vi "methodeändern-15-07-17.vi"(2 "->Methode":T2, 3 "Namen":T3) -> (1 "Methode->":T1)   [LabVIEW 2010]
panel:
  in  "T_MainMach2":dbl[](array[numeric])
  in  "t_MainMach2":dbl[](array[numeric])
  in  "T_MainMach1":dbl[](array[numeric])
  in  "t_MainMach1":dbl[](array[numeric])
  out "Methode":string
  in  "Int.Stop2":dbl
  in  "Int.Start2":dbl
  in  "Int.Stop1":dbl
  in  "Int.Start1":dbl
  in  "ZeitpktMS-2":dbl
  in  "ZeitpktMS-1":dbl
  in  "SetpointMPV":i32[](array[numeric]) min=1 max=6 step=1
  in  "ZeitpunkteMPV":dbl[](array[numeric])
  in  "Editor verlassen":bool
  out "langsameHeizungen":string[](array[string])
  out "HorstSPMod2B":string[](array[string])
  out "HorstSPMod2A":string[](array[string])
  out "HorstSPMod1":string[](array[string])
  out "HorstSPMod0":string[](array[string])
  out "DIOsSPMod0":string[](array[string])
  out "DIOsSPMod2A":string[](array[string])
  out "DIOsSPMod2B":string[](array[string])
  out "DIOsSPMod1":string[](array[string])
  in  "Zykluslängen [s]":dbl[](array[numeric])
  in  "MS-Daten?":bool
  in  "PIDs für \"träge\" Heizungen":T4(array[cluster])
  in  "T_PreMach2":dbl[](array[numeric])
  in  "t_PreMach2":dbl[](array[numeric])
  in  "T_PreMach1":dbl[](array[numeric])
  in  "t_PreMach1":dbl[](array[numeric])
  in  "FPGAFixp":dbl[][](array[numeric])
  in  "ZeitpktFPGAFixp":dbl[](array[numeric])
  in  "FPGAPID":T5(array[cluster])
  in  "ZeitpktFPGAPID":dbl[](array[numeric])
  in  "FPGABoolesch":bool[][](array[boolean])
  in  "ZPktFPGABoolesch":dbl[](array[numeric])
  in  "LHHeizen?":bool[](array[boolean])
  in  "LangsameHeizungenSP":dbl[](array[numeric])
  in  "HorstSPMod2B":dbl[][](array[numeric])
  in  "HorstSPMod2A":dbl[][](array[numeric])
  in  "HorstSPMod1":dbl[][](array[numeric])
  in  "HorstSPMod0":dbl[][](array[numeric])
  in  "Mod2BHorstZeitpkt":dbl[](array[numeric])
  in  "Mod2AHorstZeitpkt":dbl[](array[numeric])
  in  "Mod1HorstZeitpkt":dbl[](array[numeric])
  in  "Mod0HorstZeitpkt":dbl[](array[numeric])
  in  "DIOsSPMod2B":bool[][](array[boolean])
  in  "DIOsSPMod2A":bool[][](array[boolean])
  in  "DIOsSPMod1":bool[][](array[boolean])
  in  "DIOsSPMod0":bool[][](array[boolean])
  in  "ZeitpktDIOsMod2B":dbl[](array[numeric])
  in  "ZeitpktDIOsMod2A":dbl[](array[numeric])
  in  "ZeitpktDIOsMod1":dbl[](array[numeric])
  in  "ZeitpktDIOsMod0":dbl[](array[numeric])
  # "GANZ WICHTIG: ALLE TABELLEN MÜSSEN MIT DEM ZEITPUNKT 0 BEGINNEN UND DÜRFEN NICHT ENDEN, BEVOR DER ZYKLUS BEENDET IST"
  # "Alle Zeiten und Zeitpunkte werden in Sekunden ausgedrückt;\nModul0, Modul1, Modul2A, Modul2B"
  # "Schaltverhalten der Digitalausgänge, geordnet nach Modulen:\nModul0"
  # "Schaltverhalten der Digitalausgänge, geordnet nach Modulen:\nModul1"
  # "Schaltverhalten der Digitalausgänge, geordnet nach Modulen:\nModul2A"
  # "Schaltverhalten der Digitalausgänge, geordnet nach Modulen:\nModul2B"
  # "Vorgaben für die digitalen Druck-/Flußregler, geordnet nach Modulen:\nModul0"
  # "Vorgaben für die digitalen Druck-/Flußregler, geordnet nach Modulen:\nModul1"
  # "Vorgaben für die digitalen Druck-/Flußregler, geordnet nach Modulen:\nModul2A"
  # "Vorgaben für die digitalen Druck-/Flußregler, geordnet nach Modulen:\nModul2B"
  # "\"Träge\" Heizungen: PID-Werte, Temperaturvorgaben und An/Aus"
  # "Boolesche Variablen zur Steuerung von Modul1"
  # "Trap1 heizen          Trap2 heizen      PreMach1 heizen  PreMach2 heizen MainMach1 heizen MainMach2 heizen"
  # "PID-Parameter für die \"schnellen\" Heizungen"
  # "Trap1                              Trap2                            PreMach1                       PreMach2                      MainMach1                     MainMach2"
  # "Variablen zur Steuerung der \"schnellen\" Heizungen; Temperatur in °C"
  # "TSetp(Trap1)                TSetp(Trap2)"
  # "Temperaturrampen für die Vorsäulen; die eingegebenen Punkte im (t-T)-Raum werden durch lineare Funktionen verbunden, jeweils definiert von Punkt zu Punkt"
  # "Sollen die Daten vom MS abgefragt werden? Wenn ja, zu welchen Zeitpunkten (im Zyklus1)"
  # "Stellung des Multipositionsventils; die Zeitpunkte beziehen sich auf den Zyklus von Modul0.\nDie Stellungen bezeichnen: 1. Cal - 2. Span - 3. ? - 4. ? - 5. Blank - 6. Air"
  # "Innerhalb welcher Zeitfenster soll der Probenfluß integriert werden?"
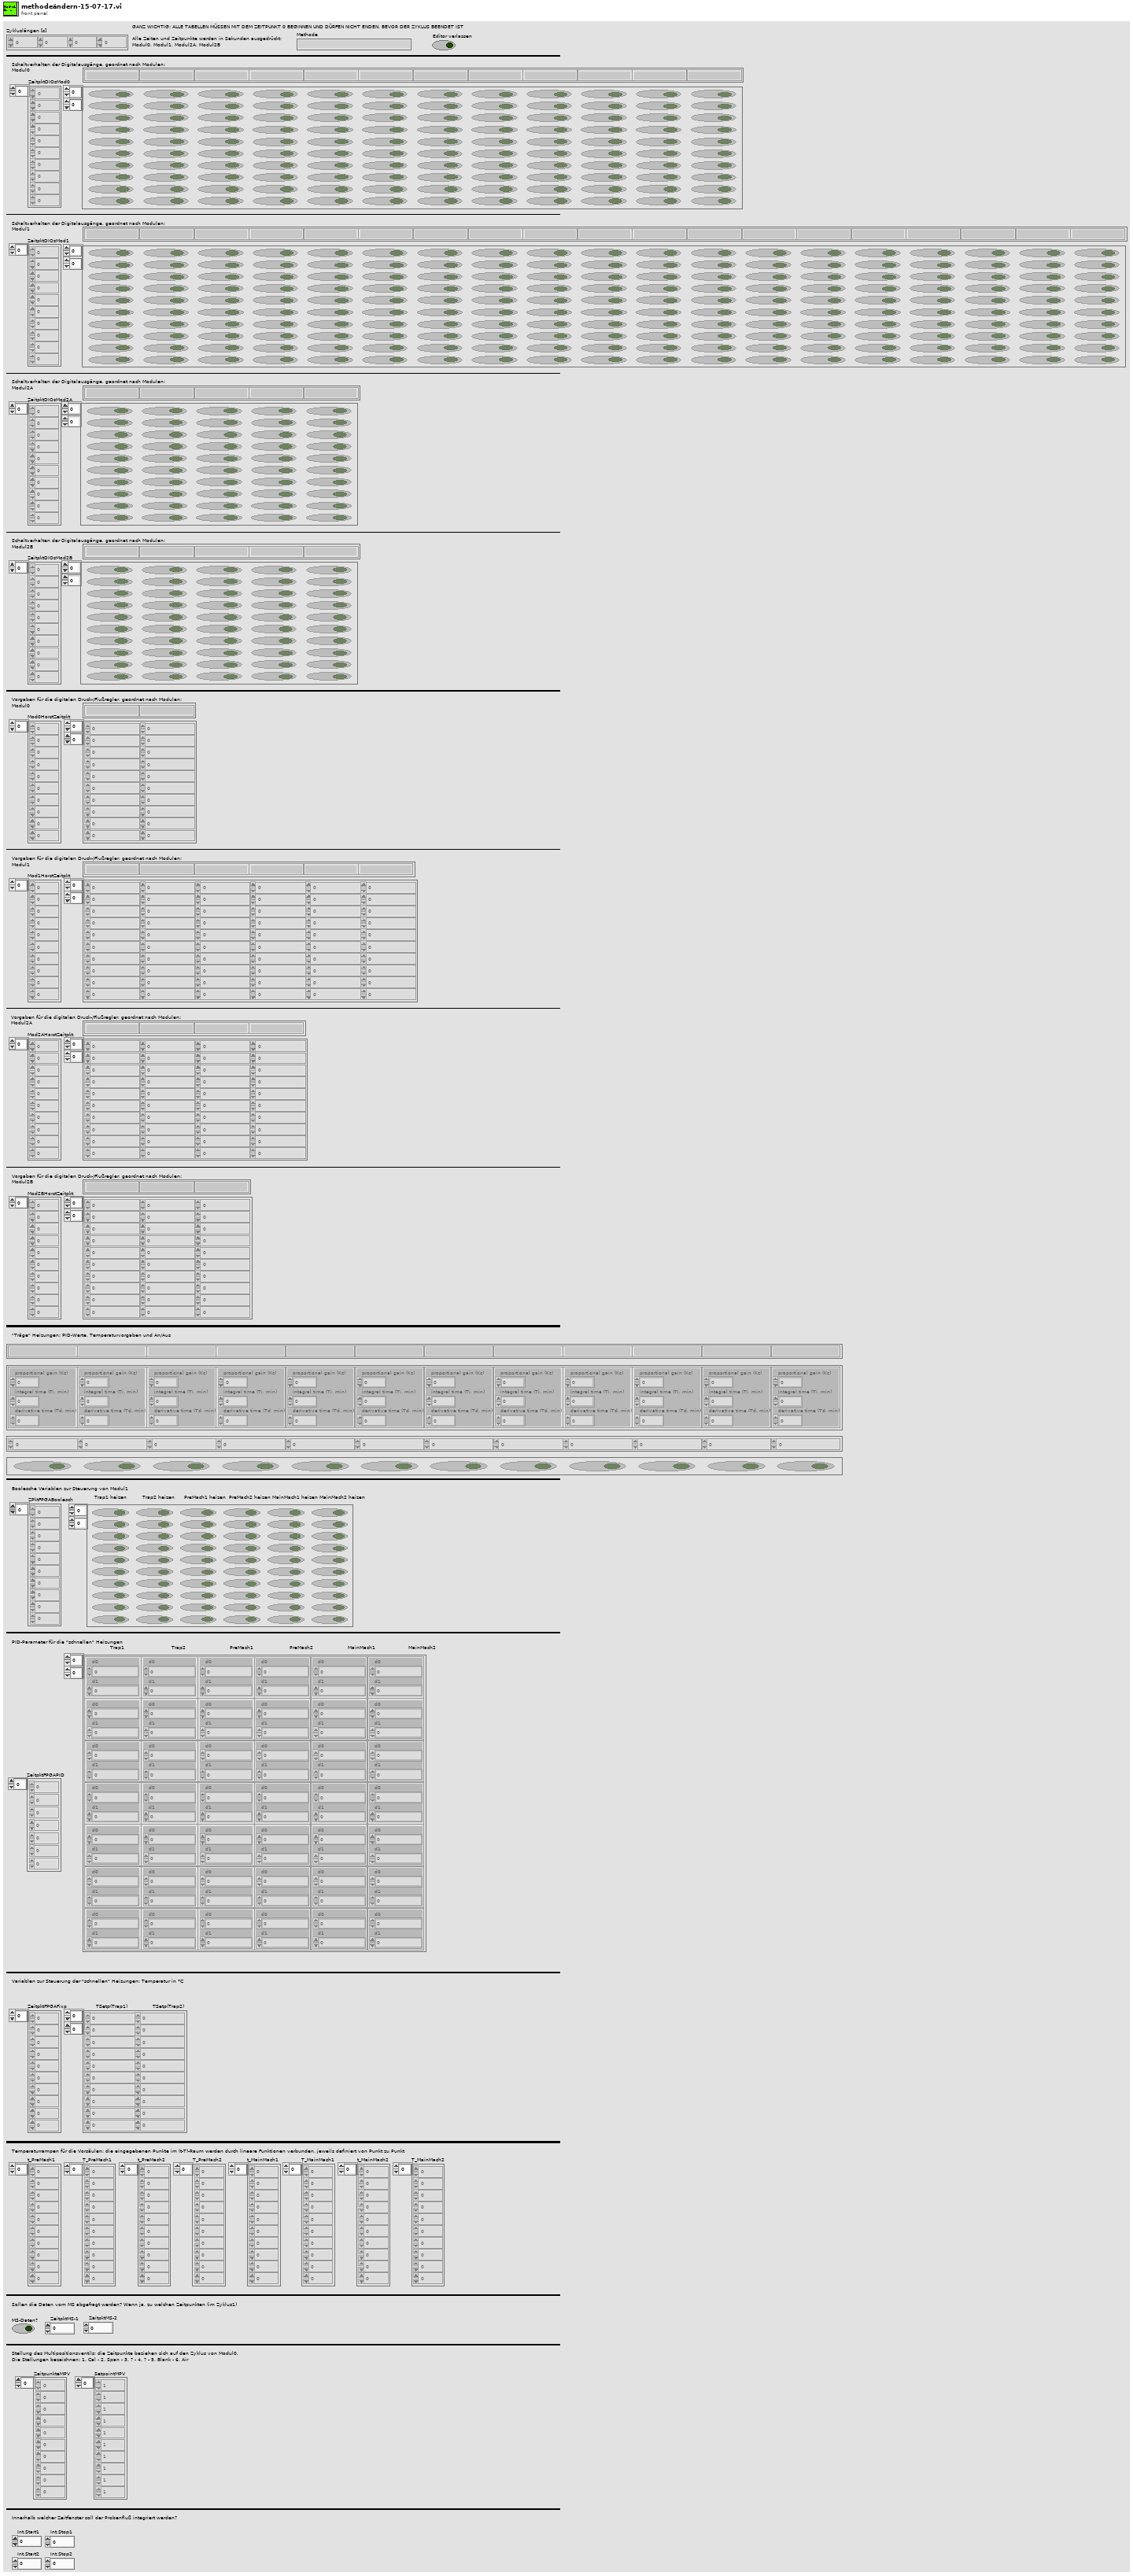
[diagram p1: front panel]
types:
  T1 = cluster{"Zykluslängen [s]":dbl[], "ZeitpktDIOsMod0":dbl[], "ZeitpktDIOsMod1":dbl[], "ZeitpktDIOsMod2A":dbl[], "ZeitpktDIOsMod2B":dbl[], "DIOsSPMod0":bool[][], "DIOsSPMod1":bool[][], "DIOsSPMod2A":bool[][], "DIOsSPMod2B":bool[][], "Mod0HorstZeitpkt":dbl[], "Mod1HorstZeitpkt":dbl[], "Mod2AHorstZeitpkt":dbl[], "Mod2BHorstZeitpkt":dbl[], "HorstSPMod0":dbl[][], "HorstSPMod1":dbl[][], "HorstSPMod2A":dbl[][], "HorstSPMod2B":dbl[][], "LangsameHeizungenSP":dbl[], "LHHeizen?":bool[], "ZPktFPGABoolesch":dbl[], "FPGABoolesch":bool[][], "ZeitpktFPGAPID":dbl[], "FPGAPID":cluster{"d0":fxp<+/-,18,18>, "d1":fxp<+/-,21,21>}[][], "ZeitpktFPGAFixp":dbl[], "FPGAFixp":dbl[][], "t_PreMach1":dbl[], "T_PreMach1":dbl[], "t_PreMach2":dbl[], "T_PreMach2":dbl[], "PIDs für \"träge\" Heizungen":cluster{"proportional gain (Kc)":dbl, "integral time (Ti, min)":dbl, "derivative time (Td, min)":dbl}[], "Zwangsbedingungen":dbl[][], "MS-Daten?":bool, "ZeitpunkteMPV":dbl[], "SetpointMPV":i32[], "ZeitpktMS-1":dbl, "ZeitpktMS-2":dbl, "Int.Start1":dbl, "Int.Stop1":dbl, "Int.Start2":dbl, "Int.Stop2":dbl, "Methodenname":string, "t_MainMach1":dbl[], "T_MainMach1":dbl[], "t_MainMach2":dbl[], "T_MainMach2":dbl[]}
  T2 = cluster{"Zykluslängen [s]":dbl[], "ZeitpktDIOsMod0":dbl[], "ZeitpktDIOsMod1":dbl[], "ZeitpktDIOsMod2A":dbl[], "ZeitpktDIOsMod2B":dbl[], "DIOsSPMod0":bool[][], "DIOsSPMod1":bool[][], "DIOsSPMod2A":bool[][], "DIOsSPMod2B":bool[][], "Mod0HorstZeitpkt":dbl[], "Mod1HorstZeitpkt":dbl[], "Mod2AHorstZeitpkt":dbl[], "Mod2BHorstZeitpkt":dbl[], "HorstSPMod0":dbl[][], "HorstSPMod1":dbl[][], "HorstSPMod2A":dbl[][], "HorstSPMod2B":dbl[][], "LHSetpoints":dbl[], "LHHeizen?":bool[], "ZPktFPGABoolesch":dbl[], "FPGABoolesch":bool[][], "ZeitpktFPGAPID":dbl[], "FPGAPID":cluster{"d0":fxp<+/-,18,18>, "d1":fxp<+/-,21,21>}[][], "ZeitpktFPGAFixp":dbl[], "SHSetpoints":dbl[][], "t_PreMach1":dbl[], "T_PreMach1":dbl[], "t_PreMach2":dbl[], "T_PreMach2":dbl[], "PIDs für \"träge\" Heizungen":cluster{"proportional gain":dbl, "integral time":dbl, "derivative time":dbl}[], "Zwangsbedingungen":dbl[][], "Dateien fürs MS schicken?":bool, "ZeitpunkteMPV":dbl[], "SPMPV":i32[], "ZeitpktMS-1":dbl, "ZeitpktMS-2":dbl, "Int.Start1":dbl, "Int.Stop1":dbl, "Int.Start2":dbl, "Int.Stop2":dbl, "Methodenname":string, "t_MainMach1":dbl[], "T_MainMach1":dbl[], "t_MainMach2":dbl[], "T_MainMach2":dbl[]}
  T3 = cluster{"DIOsMod0Name":string[], "DIOsMod1Name":string[], "DIOsMod2AName":string[], "DIOsMod2BName":string[], "HorstMod0Name":string[], "HorstMod1Name":string[], "HorstMod2AName":string[], "HorstMod2BName":string[], string[]}
  T4 = cluster{"proportional gain (Kc)":dbl, "integral time (Ti, min)":dbl, "derivative time (Td, min)":dbl}[]
  T5 = cluster{"d0":fxp<+/-,18,18>, "d1":fxp<+/-,21,21>}[][]
  T6 = cluster{"proportional gain":dbl, "integral time":dbl, "derivative time":dbl}[]
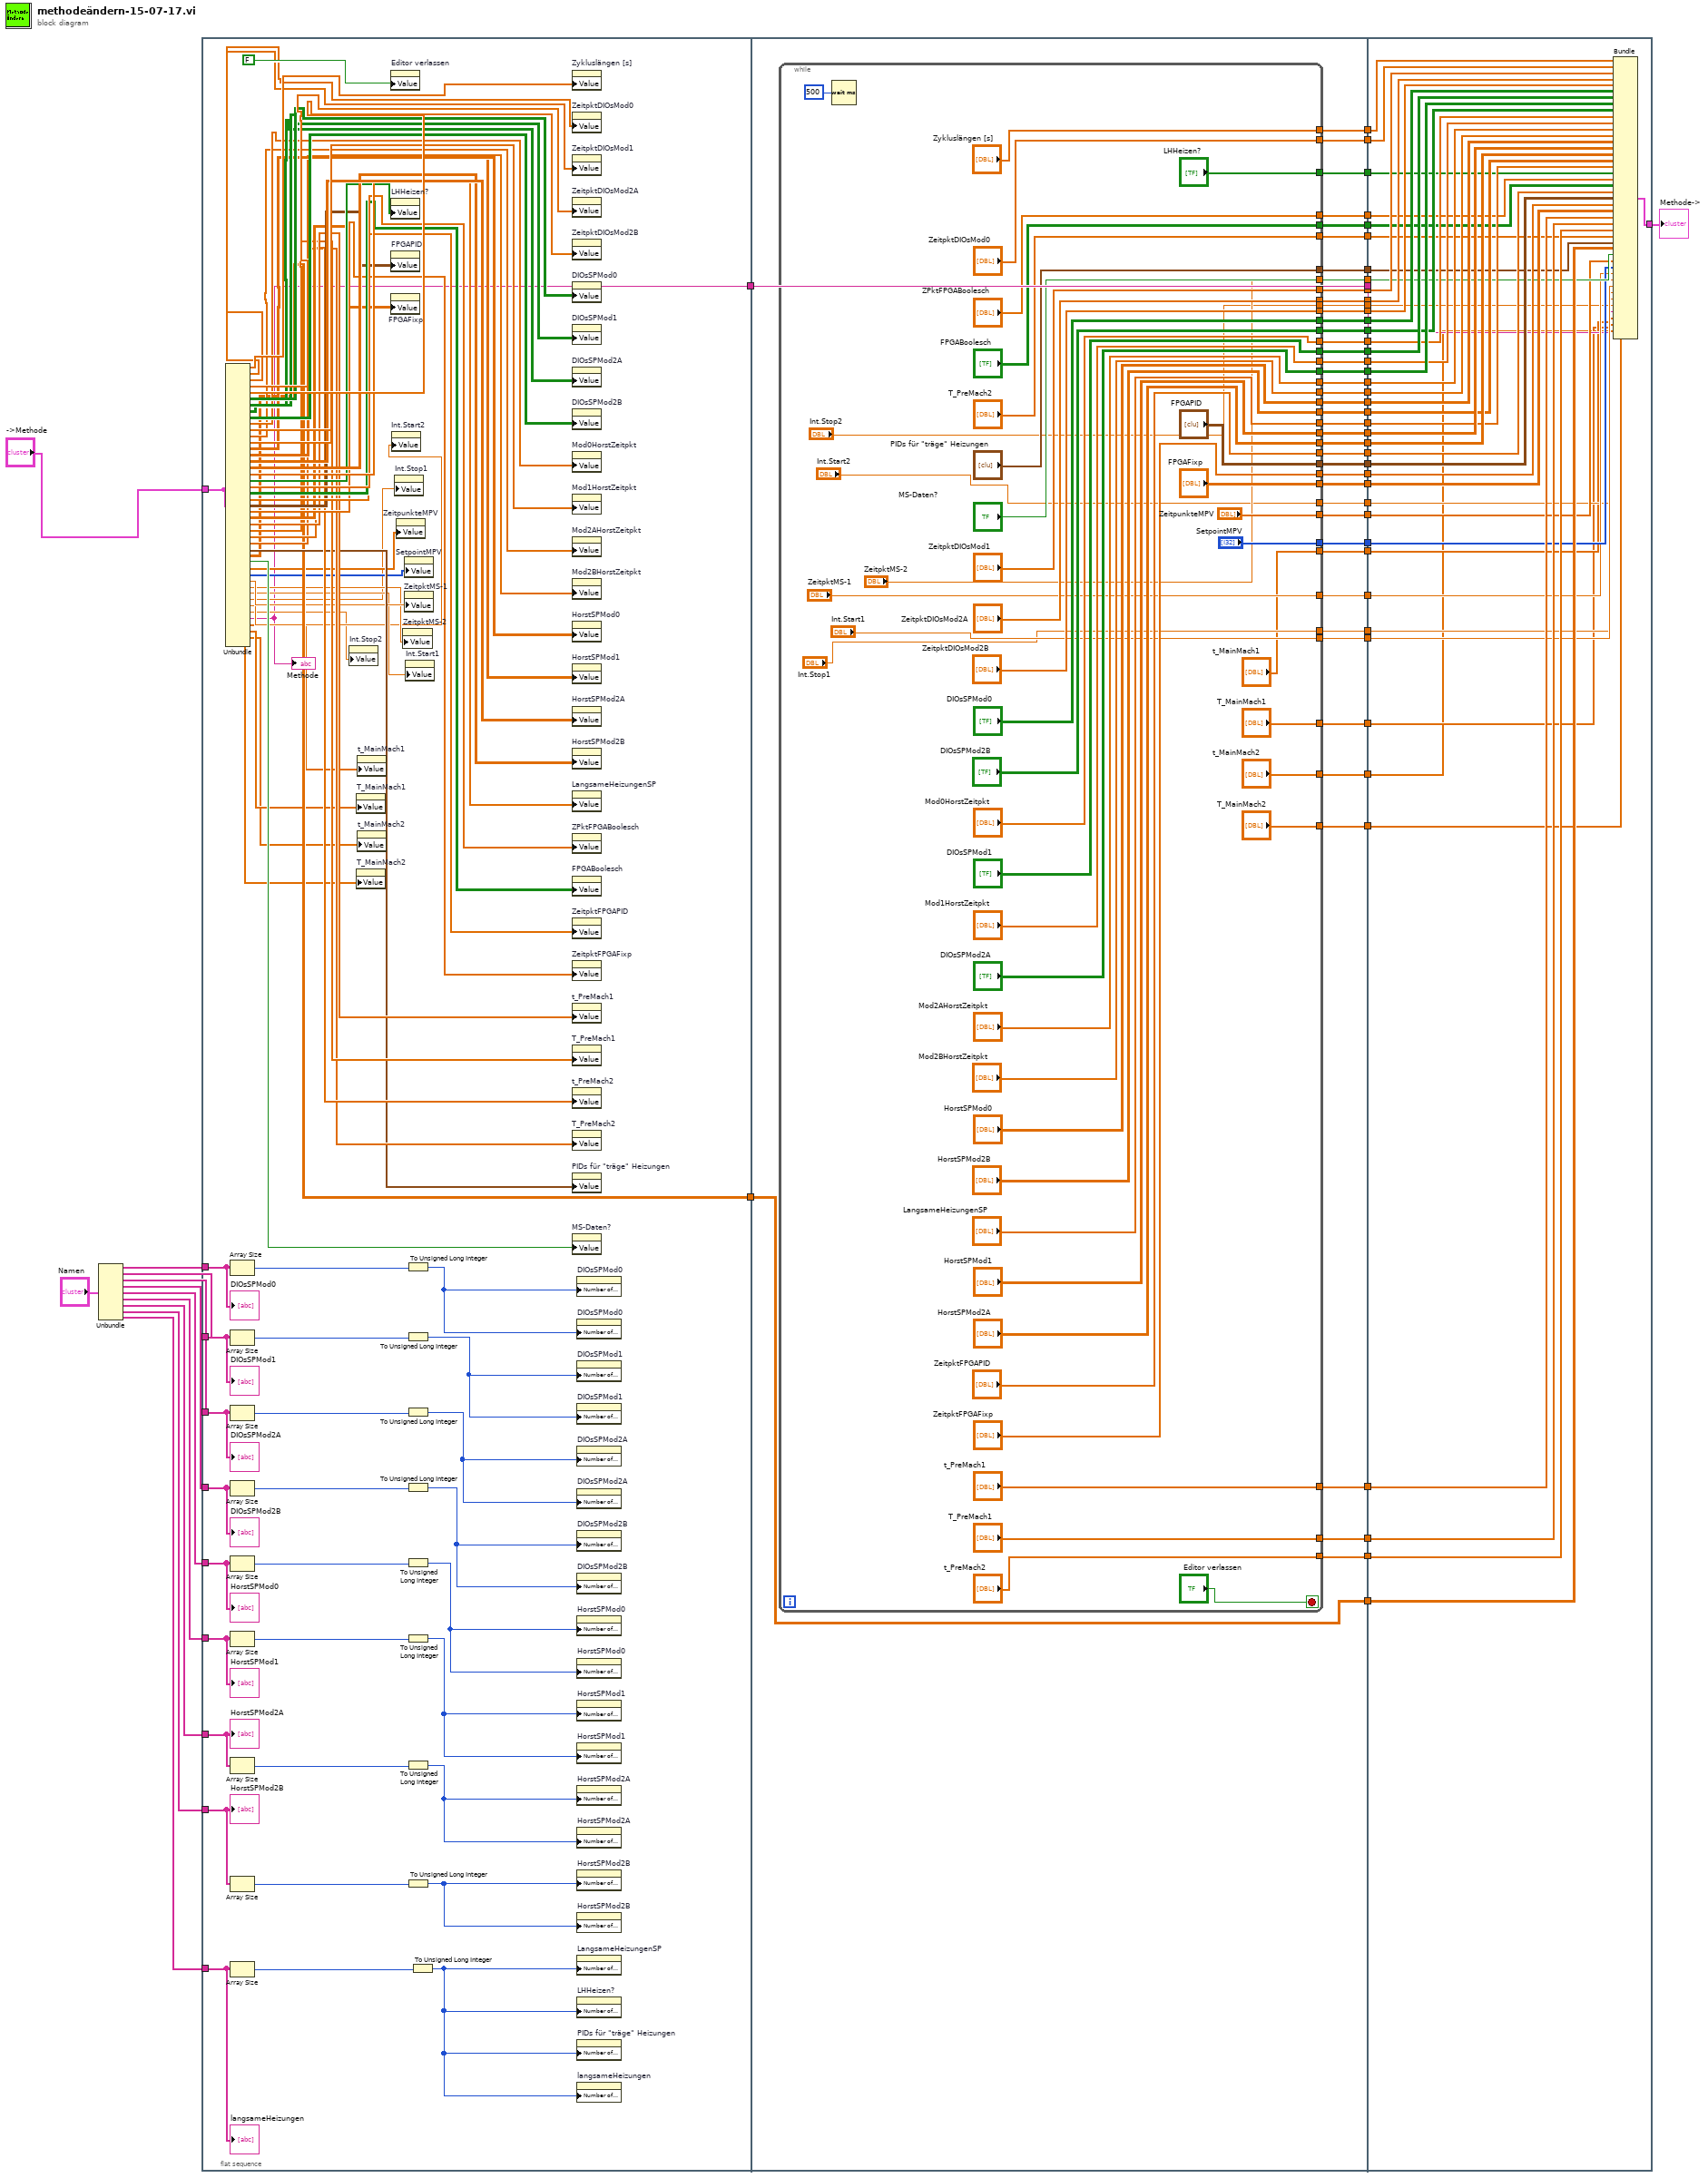
[diagram p0: block diagram]
diagram:
  n1 = Unbundle("Namen") -> ("DIOsMod0Name"=w25:string[], "DIOsMod1Name"=w24:string[], "DIOsMod2AName"=w23:string[], "DIOsMod2BName"=w22:string[], "HorstMod0Name"=w21:string[], "HorstMod1Name"=w20:string[], "HorstMod2AName"=w19:string[], "HorstMod2BName"=w18:string[], w17:string[])
  n2 = flat-sequence {
    tunnel: [w74] -> w29
    tunnel: w25 -> [w132]
    tunnel: w24 -> [w129]
    tunnel: w23 -> [w127]
    tunnel: w22 -> [w125]
    tunnel: w21 -> [w123]
    tunnel: w20 -> [w121]
    tunnel: w19 -> [w119]
    tunnel: w18 -> [w117]
    tunnel: w17 -> [w115]
    tunnel: [w105] -> _
    tunnel: "->Methode" -> [w105]
    tunnel: [w64] -> w15
    tunnel: [w178] -> w59
    tunnel: [w177] -> w58
    tunnel: [w176] -> w57
    tunnel: [w175] -> w56
    tunnel: [w174] -> w55
    tunnel: [w173] -> w54
    tunnel: [w172] -> w53
    tunnel: [w171] -> w52
    tunnel: [w170] -> w51
    tunnel: [w169] -> w50
    tunnel: [w168] -> w49
    tunnel: [w167] -> w48
    tunnel: [w166] -> w47
    tunnel: [w165] -> w46
    tunnel: [w164] -> w45
    tunnel: [w163] -> w44
    tunnel: [w162] -> w43
    tunnel: [w161] -> w42
    tunnel: [w160] -> w41
    tunnel: [w159] -> w40
    tunnel: [w158] -> w39
    tunnel: [w157] -> w38
    tunnel: [w156] -> w37
    tunnel: [w155] -> w36
    tunnel: [w154] -> w35
    tunnel: [w153] -> w34
    tunnel: [w152] -> w33
    tunnel: [w151] -> w32
    tunnel: [w150] -> w31
    tunnel: [w149] -> w30
    tunnel: w29 -> [w149]
    tunnel: [w148] -> w28
    tunnel: [w147] -> w27
    tunnel: [w146] -> w16
    tunnel: w15 -> [w146]
    tunnel: [w145] -> w14
    tunnel: [w144] -> w13
    tunnel: [w143] -> w12
    tunnel: [w142] -> w11
    tunnel: [w141] -> w10
    tunnel: [w140] -> w9
    tunnel: [w139] -> w8
    tunnel: [w138] -> w7
    tunnel: [w137] -> w6
    tunnel: [w136] -> w5
    tunnel: [w135] -> w4
    tunnel: [w134] -> w3
    tunnel: w59 -> [w269]
    tunnel: w58 -> [w268]
    tunnel: w57 -> [w267]
    tunnel: w56 -> [w266]
    tunnel: w55 -> [w265]
    tunnel: w54 -> [w264]
    tunnel: w53 -> [w263]
    tunnel: w52 -> [w262]
    tunnel: w51 -> [w261]
    tunnel: w50 -> [w260]
    tunnel: w49 -> [w259]
    tunnel: w48 -> [w258]
    tunnel: w47 -> [w257]
    tunnel: w46 -> [w256]
    tunnel: w45 -> [w255]
    tunnel: w44 -> [w254]
    tunnel: w43 -> [w253]
    tunnel: w42 -> [w252]
    tunnel: w41 -> [w251]
    tunnel: w40 -> [w250]
    tunnel: w39 -> [w249]
    tunnel: w38 -> [w248]
    tunnel: w37 -> [w247]
    tunnel: w36 -> [w246]
    tunnel: w35 -> [w245]
    tunnel: w34 -> [w244]
    tunnel: w33 -> [w243]
    tunnel: w32 -> [w242]
    tunnel: w31 -> [w241]
    tunnel: w30 -> [w240]
    tunnel: w28 -> [w238]
    tunnel: w27 -> [w239]
    tunnel: w16 -> [w228]
    tunnel: w14 -> [w237]
    tunnel: w13 -> [w236]
    tunnel: [w235] -> w1
    tunnel: w12 -> [w234]
    tunnel: w11 -> [w233]
    tunnel: w10 -> [w232]
    tunnel: w9 -> [w231]
    tunnel: w8 -> [w230]
    tunnel: w7 -> [w229]
    tunnel: w6 -> [w227]
    tunnel: w5 -> [w226]
    tunnel: w4 -> [w225]
    tunnel: w3 -> [w224]
    frame #0 {
      n3 = Unbundle(w105) -> ("Zykluslängen [s]"=w104:dbl[], "ZeitpktDIOsMod0"=w103:dbl[], "ZeitpktDIOsMod1"=w102:dbl[], "ZeitpktDIOsMod2A"=w101:dbl[], "ZeitpktDIOsMod2B"=w100:dbl[], "DIOsSPMod0"=w99:bool[][], "DIOsSPMod1"=w98:bool[][], "DIOsSPMod2A"=w97:bool[][], "DIOsSPMod2B"=w96:bool[][], "Mod0HorstZeitpkt"=w95:dbl[], "Mod1HorstZeitpkt"=w94:dbl[], "Mod2AHorstZeitpkt"=w93:dbl[], "Mod2BHorstZeitpkt"=w92:dbl[], "HorstSPMod0"=w91:dbl[][], "HorstSPMod1"=w90:dbl[][], "HorstSPMod2A"=w89:dbl[][], "HorstSPMod2B"=w88:dbl[][], "LHSetpoints"=w87:dbl[], "LHHeizen?"=w86:bool[], "ZPktFPGABoolesch"=w85:dbl[], "FPGABoolesch"=w84:bool[][], "ZeitpktFPGAPID"=w83:dbl[], "FPGAPID"=w82:T5, "ZeitpktFPGAFixp"=w81:dbl[], "SHSetpoints"=w80:dbl[][], "t_PreMach1"=w79:dbl[], "T_PreMach1"=w78:dbl[], "t_PreMach2"=w77:dbl[], "T_PreMach2"=w76:dbl[], "PIDs für \"träge\" Heizungen"=w75:T6, "Zwangsbedingungen"=w74:dbl[][], "Dateien fürs MS schicken?"=w73:bool, "ZeitpunkteMPV"=w72:dbl[], "SPMPV"=w71:i32[], "ZeitpktMS-1"=w70:dbl, "ZeitpktMS-2"=w69:dbl, "Int.Start1"=w68:dbl, "Int.Stop1"=w67:dbl, "Int.Start2"=w66:dbl, "Int.Stop2"=w65:dbl, "Methodenname"=w64:string, "t_MainMach1"=w63:dbl[], "T_MainMach1"=w62:dbl[], "t_MainMach2"=w61:dbl[], "T_MainMach2"=w60:dbl[])
      "Methode" <- w64
      n4 = Array Size(array=w132) -> (size(s)=w131:i32)
      n5 = Array Size(array=w129) -> (size(s)=w130:i32)
      n6 = Array Size(array=w127) -> (size(s)=w128:i32)
      n7 = Array Size(array=w125) -> (size(s)=w126:i32)
      n8 = Array Size(array=w123) -> (size(s)=w124:i32)
      n9 = Array Size(array=w121) -> (size(s)=w122:i32)
      n10 = Array Size(array=w119) -> (size(s)=w120:i32)
      n11 = Array Size(array=w117) -> (size(s)=w118:i32)
      n12 = Array Size(array=w115) -> (size(s)=w116:i32)
      n13 = property on="Int.Stop2" class="DigNum (strict)"("Value"=w65) -> ()  [unwired: 2 in, 2 out]
      n14 = property on="T_MainMach1" class="Arr (strict)"("Value"=w62) -> ()  [unwired: 2 in, 2 out]
      n15 = property on="T_MainMach2" class="Arr (strict)"("Value"=w60) -> ()  [unwired: 2 in, 2 out]
      n16 = property on="t_MainMach1" class="Arr (strict)"("Value"=w63) -> ()  [unwired: 2 in, 2 out]
      n17 = property on="t_MainMach2" class="Arr (strict)"("Value"=w61) -> ()  [unwired: 2 in, 2 out]
      n18 = property on="Editor verlassen" class="Bool (strict)"("Value"=FALSE) -> ()  [unwired: 2 in, 2 out]
      n19 = property on="LHHeizen?" class="Arr (strict)"("Value"=w86) -> ()  [unwired: 2 in, 2 out]
      n20 = property on="FPGAPID" class="Arr (strict)"("Value"=w82) -> ()  [unwired: 2 in, 2 out]
      n21 = property on="FPGAFixp" class="Arr (strict)"("Value"=w80) -> ()  [unwired: 2 in, 2 out]
      n22 = property on="Int.Start2" class="DigNum (strict)"("Value"=w66) -> ()  [unwired: 2 in, 2 out]
      n23 = property on="Int.Stop1" class="DigNum (strict)"("Value"=w67) -> ()  [unwired: 2 in, 2 out]
      n24 = property on="ZeitpunkteMPV" class="Arr (strict)"("Value"=w72) -> ()  [unwired: 2 in, 2 out]
      n25 = property on="ZeitpktMS-2" class="DigNum (strict)"("Value"=w69) -> ()  [unwired: 2 in, 2 out]
      n26 = property on="SetpointMPV" class="Arr (strict)"("Value"=w71) -> ()  [unwired: 2 in, 2 out]
      n27 = property on="ZeitpktMS-1" class="DigNum (strict)"("Value"=w70) -> ()  [unwired: 2 in, 2 out]
      n28 = property on="Int.Start1" class="DigNum (strict)"("Value"=w68) -> ()  [unwired: 2 in, 2 out]
      n29 = To Unsigned Long Integer(number=w131) -> (unsigned 32bit integer=w114:u32)
      n30 = To Unsigned Long Integer(number=w130) -> (unsigned 32bit integer=w113:u32)
      n31 = To Unsigned Long Integer(number=w128) -> (unsigned 32bit integer=w112:u32)
      n32 = To Unsigned Long Integer(number=w126) -> (unsigned 32bit integer=w111:u32)
      n33 = To Unsigned Long Integer(number=w124) -> (unsigned 32bit integer=w110:u32)
      n34 = To Unsigned Long Integer(number=w122) -> (unsigned 32bit integer=w109:u32)
      n35 = To Unsigned Long Integer(number=w120) -> (unsigned 32bit integer=w108:u32)
      n36 = To Unsigned Long Integer(number=w118) -> (unsigned 32bit integer=w107:u32)
      n37 = To Unsigned Long Integer(number=w116) -> (unsigned 32bit integer=w106:u32)
      n38 = property on="Zykluslängen [s]" class="Arr (strict)"("Value"=w104) -> ()  [unwired: 2 in, 2 out]
      n39 = property on="ZeitpktDIOsMod0" class="Arr (strict)"("Value"=w103) -> ()  [unwired: 2 in, 2 out]
      n40 = property on="ZeitpktDIOsMod1" class="Arr (strict)"("Value"=w102) -> ()  [unwired: 2 in, 2 out]
      n41 = property on="ZeitpktDIOsMod2A" class="Arr (strict)"("Value"=w101) -> ()  [unwired: 2 in, 2 out]
      n42 = property on="ZeitpktDIOsMod2B" class="Arr (strict)"("Value"=w100) -> ()  [unwired: 2 in, 2 out]
      n43 = property on="DIOsSPMod0" class="Arr (strict)"("Value"=w99) -> ()  [unwired: 2 in, 2 out]
      n44 = property on="DIOsSPMod1" class="Arr (strict)"("Value"=w98) -> ()  [unwired: 2 in, 2 out]
      n45 = property on="DIOsSPMod2A" class="Arr (strict)"("Value"=w97) -> ()  [unwired: 2 in, 2 out]
      n46 = property on="DIOsSPMod2B" class="Arr (strict)"("Value"=w96) -> ()  [unwired: 2 in, 2 out]
      n47 = property on="Mod0HorstZeitpkt" class="Arr (strict)"("Value"=w95) -> ()  [unwired: 2 in, 2 out]
      n48 = property on="Mod1HorstZeitpkt" class="Arr (strict)"("Value"=w94) -> ()  [unwired: 2 in, 2 out]
      n49 = property on="Mod2AHorstZeitpkt" class="Arr (strict)"("Value"=w93) -> ()  [unwired: 2 in, 2 out]
      n50 = property on="Mod2BHorstZeitpkt" class="Arr (strict)"("Value"=w92) -> ()  [unwired: 2 in, 2 out]
      n51 = property on="HorstSPMod0" class="Arr (strict)"("Value"=w91) -> ()  [unwired: 2 in, 2 out]
      n52 = property on="HorstSPMod1" class="Arr (strict)"("Value"=w90) -> ()  [unwired: 2 in, 2 out]
      n53 = property on="HorstSPMod2A" class="Arr (strict)"("Value"=w89) -> ()  [unwired: 2 in, 2 out]
      n54 = property on="HorstSPMod2B" class="Arr (strict)"("Value"=w88) -> ()  [unwired: 2 in, 2 out]
      n55 = property on="LangsameHeizungenSP" class="Arr (strict)"("Value"=w87) -> ()  [unwired: 2 in, 2 out]
      n56 = property on="ZPktFPGABoolesch" class="Arr (strict)"("Value"=w85) -> ()  [unwired: 2 in, 2 out]
      n57 = property on="FPGABoolesch" class="Arr (strict)"("Value"=w84) -> ()  [unwired: 2 in, 2 out]
      n58 = property on="ZeitpktFPGAPID" class="Arr (strict)"("Value"=w83) -> ()  [unwired: 2 in, 2 out]
      n59 = property on="ZeitpktFPGAFixp" class="Arr (strict)"("Value"=w81) -> ()  [unwired: 2 in, 2 out]
      n60 = property on="t_PreMach1" class="Arr (strict)"("Value"=w79) -> ()  [unwired: 2 in, 2 out]
      n61 = property on="T_PreMach1" class="Arr (strict)"("Value"=w78) -> ()  [unwired: 2 in, 2 out]
      n62 = property on="t_PreMach2" class="Arr (strict)"("Value"=w77) -> ()  [unwired: 2 in, 2 out]
      n63 = property on="T_PreMach2" class="Arr (strict)"("Value"=w76) -> ()  [unwired: 2 in, 2 out]
      n64 = property on="PIDs für \"träge\" Heizungen" class="Arr (strict)"("Value"=w75) -> ()  [unwired: 2 in, 2 out]
      n65 = property on="MS-Daten?" class="Bool (strict)"("Value"=w73) -> ()  [unwired: 2 in, 2 out]
      n66 = property on="DIOsSPMod0" class="Arr (strict)"("Number of Columns"=w114) -> ()  [unwired: 2 in, 2 out]
      n67 = property on="DIOsSPMod0" class="Arr (strict)"("Number of Columns"=w114) -> ()  [unwired: 2 in, 2 out]
      n68 = property on="DIOsSPMod1" class="Arr (strict)"("Number of Columns"=w113) -> ()  [unwired: 2 in, 2 out]
      n69 = property on="DIOsSPMod1" class="Arr (strict)"("Number of Columns"=w113) -> ()  [unwired: 2 in, 2 out]
      n70 = property on="DIOsSPMod2A" class="Arr (strict)"("Number of Columns"=w112) -> ()  [unwired: 2 in, 2 out]
      n71 = property on="DIOsSPMod2A" class="Arr (strict)"("Number of Columns"=w112) -> ()  [unwired: 2 in, 2 out]
      n72 = property on="DIOsSPMod2B" class="Arr (strict)"("Number of Columns"=w111) -> ()  [unwired: 2 in, 2 out]
      n73 = property on="DIOsSPMod2B" class="Arr (strict)"("Number of Columns"=w111) -> ()  [unwired: 2 in, 2 out]
      n74 = property on="HorstSPMod0" class="Arr (strict)"("Number of Columns"=w110) -> ()  [unwired: 2 in, 2 out]
      n75 = property on="HorstSPMod0" class="Arr (strict)"("Number of Columns"=w110) -> ()  [unwired: 2 in, 2 out]
      n76 = property on="HorstSPMod1" class="Arr (strict)"("Number of Columns"=w109) -> ()  [unwired: 2 in, 2 out]
      n77 = property on="HorstSPMod1" class="Arr (strict)"("Number of Columns"=w109) -> ()  [unwired: 2 in, 2 out]
      n78 = property on="HorstSPMod2A" class="Arr (strict)"("Number of Columns"=w108) -> ()  [unwired: 2 in, 2 out]
      n79 = property on="HorstSPMod2A" class="Arr (strict)"("Number of Columns"=w108) -> ()  [unwired: 2 in, 2 out]
      n80 = property on="HorstSPMod2B" class="Arr (strict)"("Number of Columns"=w107) -> ()  [unwired: 2 in, 2 out]
      n81 = property on="HorstSPMod2B" class="Arr (strict)"("Number of Columns"=w107) -> ()  [unwired: 2 in, 2 out]
      n82 = property on="LangsameHeizungenSP" class="Arr (strict)"("Number of Columns"=w106) -> ()  [unwired: 2 in, 2 out]
      n83 = property on="LHHeizen?" class="Arr (strict)"("Number of Columns"=w106) -> ()  [unwired: 2 in, 2 out]
      n84 = property on="PIDs für \"träge\" Heizungen" class="Arr (strict)"("Number of Columns"=w106) -> ()  [unwired: 2 in, 2 out]
      n85 = property on="langsameHeizungen" class="Arr (strict)"("Number of Columns"=w106) -> ()  [unwired: 2 in, 2 out]
      "DIOsSPMod1" <- w129
      "DIOsSPMod2B" <- w125
      "DIOsSPMod2A" <- w127
      "DIOsSPMod0" <- w132
      "HorstSPMod0" <- w123
      "HorstSPMod1" <- w121
      "HorstSPMod2A" <- w119
      "HorstSPMod2B" <- w117
      "langsameHeizungen" <- w115
    }
    frame #1 {
      n86 = while {
        tunnel: ["ZeitpktDIOsMod0"] -> w178
        tunnel: ["ZeitpktDIOsMod1"] -> w177
        tunnel: ["ZeitpktDIOsMod2A"] -> w176
        tunnel: ["ZeitpktDIOsMod2B"] -> w175
        tunnel: ["DIOsSPMod0"] -> w174
        tunnel: ["DIOsSPMod1"] -> w173
        tunnel: ["DIOsSPMod2A"] -> w172
        tunnel: ["DIOsSPMod2B"] -> w171
        tunnel: ["Mod0HorstZeitpkt"] -> w170
        tunnel: ["Mod1HorstZeitpkt"] -> w169
        tunnel: ["Mod2AHorstZeitpkt"] -> w168
        tunnel: ["Mod2BHorstZeitpkt"] -> w167
        tunnel: ["HorstSPMod0"] -> w166
        tunnel: ["HorstSPMod1"] -> w165
        tunnel: ["HorstSPMod2A"] -> w164
        tunnel: ["HorstSPMod2B"] -> w163
        tunnel: ["LangsameHeizungenSP"] -> w162
        tunnel: ["LHHeizen?"] -> w161
        tunnel: ["ZPktFPGABoolesch"] -> w160
        tunnel: ["FPGABoolesch"] -> w159
        tunnel: ["ZeitpktFPGAPID"] -> w158
        tunnel: ["FPGAPID"] -> w157
        tunnel: ["ZeitpktFPGAFixp"] -> w156
        tunnel: ["FPGAFixp"] -> w155
        tunnel: ["t_PreMach1"] -> w154
        tunnel: ["T_PreMach1"] -> w153
        tunnel: ["t_PreMach2"] -> w152
        tunnel: ["T_PreMach2"] -> w151
        tunnel: ["PIDs für \"träge\" Heizungen"] -> w150
        tunnel: ["MS-Daten?"] -> w148
        tunnel: ["Zykluslängen [s]"] -> w147
        tunnel: ["ZeitpunkteMPV"] -> w145
        tunnel: ["SetpointMPV"] -> w144
        tunnel: ["ZeitpktMS-1"] -> w143
        tunnel: ["ZeitpktMS-2"] -> w142
        tunnel: ["Int.Start1"] -> w141
        tunnel: ["Int.Stop1"] -> w140
        tunnel: ["Int.Start2"] -> w139
        tunnel: ["Int.Stop2"] -> w138
        tunnel: ["t_MainMach1"] -> w137
        tunnel: ["T_MainMach1"] -> w136
        tunnel: ["t_MainMach2"] -> w135
        tunnel: ["T_MainMach2"] -> w134
        stop <- "Editor verlassen" stop-if-true
        n87 = Wait (ms)(milliseconds to wait=u32 500 ("Zu wartende ms")) -> ()  [unwired: 1 out]
      }
    }
    frame #2 {
      n88 = Bundle("Zykluslängen [s]"=w239, "ZeitpktDIOsMod0"=w269, "ZeitpktDIOsMod1"=w268, "ZeitpktDIOsMod2A"=w267, "ZeitpktDIOsMod2B"=w266, "DIOsSPMod0"=w265, "DIOsSPMod1"=w264, "DIOsSPMod2A"=w263, "DIOsSPMod2B"=w262, "Mod0HorstZeitpkt"=w261, "Mod1HorstZeitpkt"=w260, "Mod2AHorstZeitpkt"=w259, "Mod2BHorstZeitpkt"=w258, "HorstSPMod0"=w257, "HorstSPMod1"=w256, "HorstSPMod2A"=w255, "HorstSPMod2B"=w254, "LangsameHeizungenSP"=w253, "LHHeizen?"=w252, "ZPktFPGABoolesch"=w251, "FPGABoolesch"=w250, "ZeitpktFPGAPID"=w249, "FPGAPID"=w248, "ZeitpktFPGAFixp"=w247, "FPGAFixp"=w246, "t_PreMach1"=w245, "T_PreMach1"=w244, "t_PreMach2"=w243, "T_PreMach2"=w242, "PIDs für \"träge\" Heizungen"=w241, "Zwangsbedingungen"=w240, "MS-Daten?"=w238, "ZeitpunkteMPV"=w237, "SetpointMPV"=w236, "ZeitpktMS-1"=w234, "ZeitpktMS-2"=w233, "Int.Start1"=w232, "Int.Stop1"=w231, "Int.Start2"=w230, "Int.Stop2"=w229, "Methodenname"=w228, "t_MainMach1"=w227, "T_MainMach1"=w226, "t_MainMach2"=w225, "T_MainMach2"=w224) -> (w235:T1)  [unwired: 1 in]
    }
  }
  "Methode->" <- w1
